vi "PH_Stepmotor_BaseClass.Evt Call Relative Move.vi"(0 "i ref in":refnum<vi>, 1 "Address":T2={"Instance"="N/A", "Motor Nr"=0}, 4 "direction":T1, 5 "error in":errorcluster) -> (14 "i ref out":refnum<vi>, 19 "error out":errorcluster)   [LabVIEW 2014, in "PH_Stepmotor_BaseClass.lvlib"]
uses:
  PH_Stepmotor_BaseClass.lvlib
  PH_Stepmotor_BaseClass.Axis Address.ctl
  PH_Stepmotor_BaseClass.Axis Direction.ctl
  CS_Core/CSSystem/CoreLib/CoreLib.short 2 byte array.vi
  CS_Core/CSSystem/CoreLib/CoreLib.int 2 byte array.vi
  CS_Core/CSSystem/CoreLib/CoreLib.lvlib
  CS_Core/BaseProcess/BaseProcess.lvlib
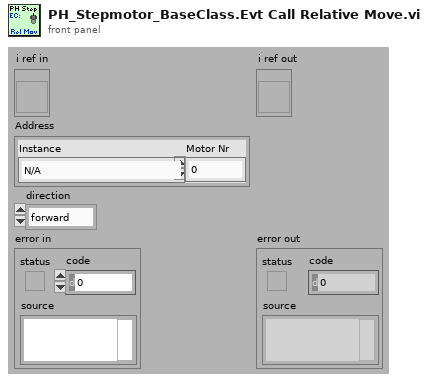
[diagram p1: front panel]
types:
  T1 = typedef "PH_Stepmotor_BaseClass.lvlib/PH_Stepmotor_BaseClass.Axis Direction.ctl" = enum16{"forward", "backward"}
  T2 = typedef "PH_Stepmotor_BaseClass.lvlib/PH_Stepmotor_BaseClass.Axis Address.ctl" = cluster{"Instance":string, "Motor Nr":i32}
  T3 = typedef "CoreDefs.rawDataType.ctl" = i8[]
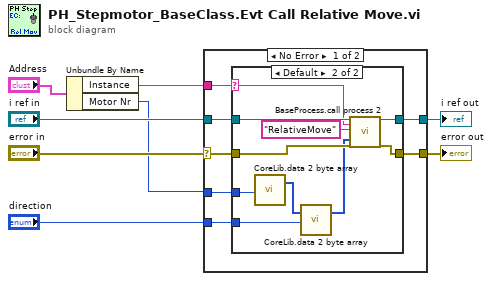
[diagram p0: block diagram]
diagram:
  n1 = Unbundle By Name("Address") -> ("Instance"=w2:string, "Motor Nr"=w1:i32)
  n2 = case shown="No Error" "error in" {
    selector: "error in" -> [w11 w28]
    tunnel: [w15 w28] -> w5
    tunnel: w2 -> [w10 _]
    tunnel: "i ref in" -> [w14 w29]
    tunnel: [w13 w29] -> w7
    tunnel: w1 -> [w12 _]
    tunnel: "direction" -> [w9 _]
    frame No Error {
      n3 = case shown="Default" w10 {
        selector: w10 -> [_ w18]
        tunnel: [w17 w27] -> w15
        tunnel: w11 -> [w17 w25]
        tunnel: w14 -> [w16 w24]
        tunnel: [w16 w23] -> w13
        tunnel: w12 -> [_ w22]
        tunnel: w9 -> [_ w20]
        frame "N/A" {
        }
        frame Default {
          n4 = call-poly "CoreLib.data 2 byte array.vi"("i32"=w22) -> ("byteArray out"=w21:T3)  [unwired: 18 in]
          n5 = call-poly "CoreLib.data 2 byte array.vi"("byteArray"=w21, "i16"=w20) -> ("byteArray out"=w19:T3)  [unwired: 17 in]
          n6 = call "BaseProcess.call process 2.vi"("i ref in"=w24, "Object"=w18, "Selector"="RelativeMove", "Data"=w19, "error in (no error)"=w25) -> ("i ref out"=w23:refnum<vi>, "error out"=w27:errorcluster)  [unwired: 13 in]
        }
      }
    }
    frame Error {
    }
  }
  "i ref out" <- w7
  "error out" <- w5
